vi "Square Function.vi"(1 "x":dbl format="%0.2f") -> (0 "square(x)":dbl format="%0.2f")   [LabVIEW 2009]
doc: "Generates the square function for any real number <B>x</B>."
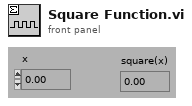
[diagram p1: front panel]
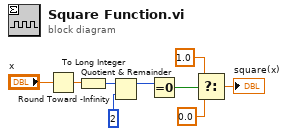
[diagram p0: block diagram]
diagram:
  n1 = Round Toward -Infinity(1:"x") -> (0:w5:dbl)
  n2 = To Long Integer(number=w5) -> (32bit integer=w4:i32)
  n3 = Quotient & Remainder(x=w4, y=2) -> (x-y*floor(x/y)=w2:i32)  [unwired: 1 out]
  n4 = Equal To 0?(x=w2) -> (x = 0?=w1:bool)
  n5 = Select(t=1.0, s=w1, f=0.0) -> (s? t:f=→"square(x)":dbl)
